vi "ReadReadoutTime.vi"(0 "object in":refnum<class "Hamamatsu.lvclass">, 5 "error in (no error)":errorcluster) -> (14 "object out":refnum<class "Hamamatsu.lvclass">, 16 "ReadoutTime":dbl, 19 "error out":errorcluster)   [LabVIEW 2021, in "Hamamatsu.lvclass"]
uses:
  Hamamatsu.lvclass
  Hamamatsu.lvclass/Hamamatsu.ctl
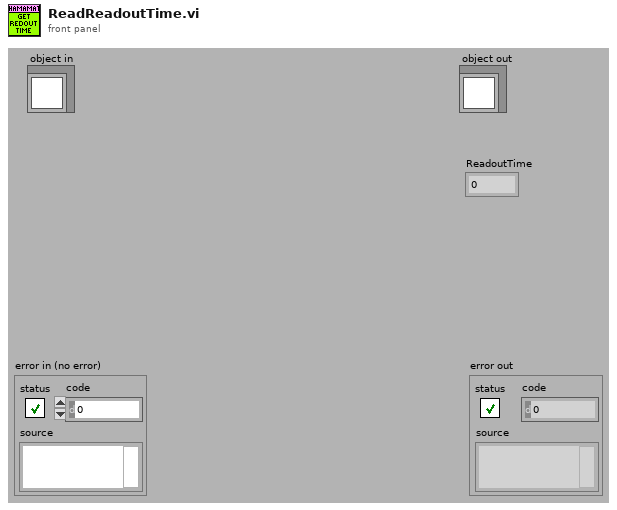
[diagram p1: front panel]
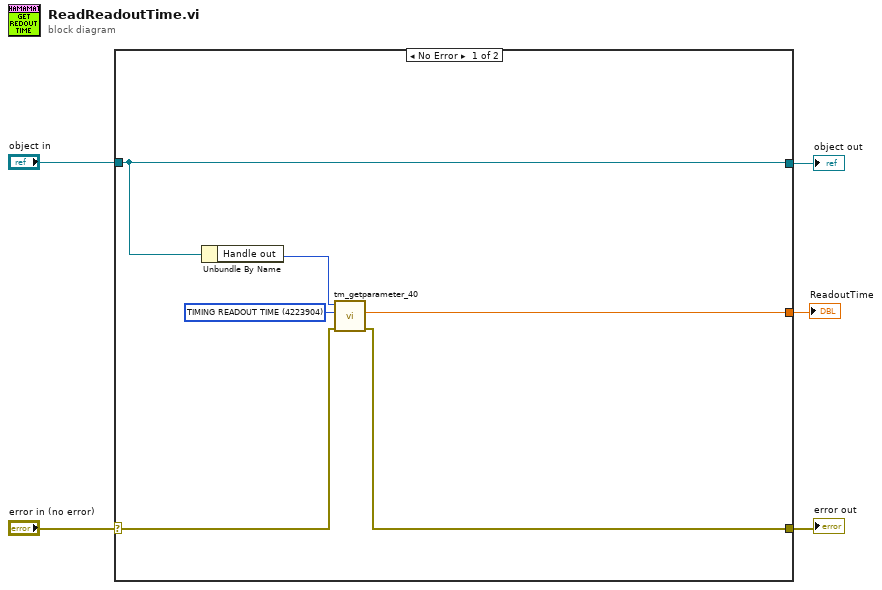
[diagram p0: block diagram]
diagram:
  n1 = case shown="No Error" "error in (no error)" {
    selector: "error in (no error)" -> [w8 w13]
    tunnel: [w7 w13] -> w4
    tunnel: [w11 w12] -> w2
    tunnel: "object in" -> [w11 w12]
    tunnel: [w6 _] -> w1
    frame No Error {
      w9 = u32 4223904 items=["SENSOR MODE"=4212128, "SENSOR MODE LINE BUNDLE HEIGHT"=4212192, "READOUT DIRECTION"=4211904, "BIT PER CHANNEL"=4342976, "EXPOSURE TIME"=2049184, "CONTRAST GAIN"=3163312, "BINNING"=4215968, "TIMING READOUT TIME"=4223904, "INTERNAL FRAME RATE"=4225952, "INTERNAL FRAME INTERVAL"=4225968, "INTERNAL LINE SPEED"=4226000, "IMAGE WIDTH"=4343200, "IMAGE HEIGHT"=4343216, "IMAGE ROWBYTES"=4343232, "IMAGE FRAMEBYTES"=4343248, "IMAGE PIXEL TYPE"=4343296] ("Parameter")
      n2 = Unbundle By Name(w11) -> ("Handle out"=w10:u32)
      n3 = call <userlib>:"tm_getparameter_40.vi"("error in (no error)"=w8, "Parameter"=w9, "Handle in"=w10) -> ("error out"=w7:errorcluster, "Value out"=w6:dbl)  [unwired: 6 in, 1 out]
    }
    frame Error {
    }
  }
  "error out" <- w4
  "object out" <- w2
  "ReadoutTime" <- w1
